vi "LuaVIEW Pull (I16).vi"(5 "LuaVIEW reference in":T1, 11 "error in (no error)":errorcluster) -> (4 "I16":i16, 6 "LuaVIEW reference out":T1, 15 "error out":errorcluster)   [LabVIEW 2013]
doc: "Retrieves an I16 data item from the head/bottom of the Lua stack and removes it, thereby shifting any remaining data items down by one. This VI is part of a polymorphic set that supports the pulling various data types. To change the type being pulled, pop up on this VI's diagram icon and use the \"Select Type\" sub menu."
uses:
  typedefs/t_LuaVIEW Reference.ctl
  typedefs/et_LuaVIEW CIN Actions.ctl
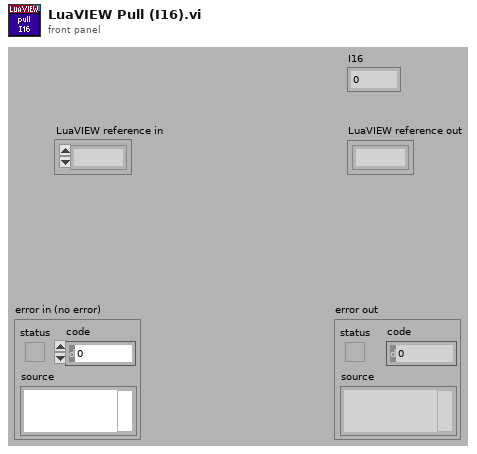
[diagram p1: front panel]
types:
  T1 = typedef "t_LuaVIEW Reference.ctl" = refnum<k1>
  T2 = typedef "et_LuaVIEW CIN Actions.ctl" = enum16{"checksynopsis", "_open", "_registerpublic", "_registerexport", "__never_an_error_result_ns", "luaversion", "cinversion", "_totals", "_taskcount", "pathological", "_unregnextpublic", "registryusecount", "__per_state_actions", "regsetprivate", "regsetindex", "regsetmodule", "_revokeexports", "_usepublic", "prepare", "compile", "execute", "call", "unregstaterefs", "_close", "pullboolean", "pullnumber", "pullI8", "pullU8", "pullI16", "pullU16", "pullI32", "pullU32", "pullobject", "pullrefnum", "pullstring", "pullflat", "pushflat", "pushobject", "getattribute", "setattribute", "stacktostring", "_startyieldtest", "_endyieldtest", "_pollprintbuffer", "__never_an_error_result_ps", "_pollexport", "setclone", "forcecleanup", "gettop", "clearstack", "insert", "pushboolean", "pushnumber", "pushrefnum", "pushstring", "pushnil", "pushvalue", "gettaskref", "settaskref"}
  T3 = typedef "et_LuaVIEW CIN Results.ctl" = enum16{"OK", "error", "main", "call", "clonecall", "modulecall", "exportcall", "index", "yield"}
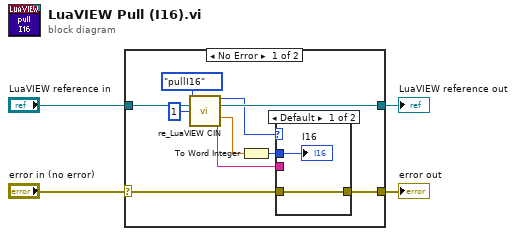
[diagram p0: block diagram]
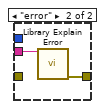
[diagram p2: hidden frame]
diagram:
  n1 = case shown="No Error" "error in (no error)" {
    selector: "error in (no error)" -> [w9 w20]
    tunnel: [w11 w19] -> w1
    tunnel: [w10 w20] -> w2
    tunnel: "LuaVIEW reference in" -> [w13 w19]
    frame No Error {
      n2 = call "re_LuaVIEW CIN.vi"("action"=et_LuaVIEW_CIN_Actions."pullI16", "LuaVIEW reference in"=w13, "index in"=1) -> ("result"=w8:T3, "LuaVIEW reference out"=w11:T1, "number out"=w6:dbl, "string out"=w7:string)  [unwired: 6 in, 3 out]
      n3 = To Word Integer(number=w6) -> (16bit integer=w5:i16)
      n4 = case shown="Default" w8 {
        tunnel: w7 -> [_ w18]
        tunnel: [w16 w17] -> w10
        tunnel: w9 -> [w16 _]
        tunnel: w5 -> [w15 _]
        frame Default {
          "I16" <- w15
        }
        frame "error" {
          n5 = call "Library Explain Error.vi"("explanation prefix (none)"=w18) -> ("explained error"=w17:errorcluster)  [unwired: 14 in]
        }
      }
    }
    frame Error {
    }
  }
  "LuaVIEW reference out" <- w1
  "error out" <- w2
